vi "Get_Num_actortype.vi"(11 "Type":string) -> (3 "Type count":i32)   [LabVIEW 2010]
doc: "This Vi implements the routine for getting the number of actors of the specified type that are running in memory.\n\nCreated by Davis Montenegro\nEPRI\n06-23-2017"
uses:
  Vars/Comm_Vars.vi
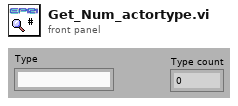
[diagram p1: front panel]
types:
  T1 = cluster{"actor_name":string, "actor_type":string, "queue":variant}[]
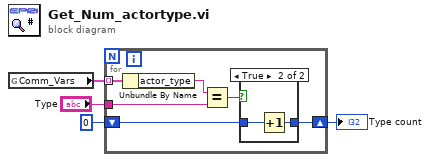
[diagram p0: block diagram]
diagram:
  n1 = global read "Comm_Vars.vi" "Comm_Vars"() -> (w4:T1)
  n2 = for {
    tunnel: w4 -> [w10] mode=indexing
    tunnel: "Type" -> [w9]
    shift-right: [w5] -> w1
    shift-left: 0 -> [w6]
    n3 = Unbundle By Name(w10) -> ("actor_type"=w8:string)
    n4 = Equal?(x=w8, y=w9) -> (x = y?=w7:bool)
    n5 = case shown="True" w7 {
      tunnel: w6 -> [w11 w13]
      tunnel: [w11 w12] -> w5
      frame False {
      }
      frame True {
        n6 = Increment(x=w13) -> (x+1=w12:i32)
      }
    }
  }
  "Type count" <- w1
